vi "PCO_SetRecordingStruct.vi"(8 "error in (no error)":errorcluster {"code" format="%x"}, 10 "strRecording":T1, 11 "ph":u64) -> (0 "error out":errorcluster {"code" format="%x"}, 2 "ErrorMessage":i32 format="%x", 3 "ph out":u64)   [LabVIEW 2019, in "SDK.lvlib" / "RecordingControl.lvlib"]
doc: "<b>Description:</b>\nThis function does set the complete set of recording settings at once. For the sake of clarity it is better to use the functions which change distinct parameter despite changing all settings at once.\nAn invalid value for one of the parameter will result in a failure response message.\nThe command will be rejected, if Recording State is [run], see PCO_GetRecordingState.\n\n<b>Supported camera type:</b>\nAll cameras\n\n<b>Descriptor dependency:</b>\nNone"
uses:
  RecordingControl.lvlib
  Structures/Structures.lvlib
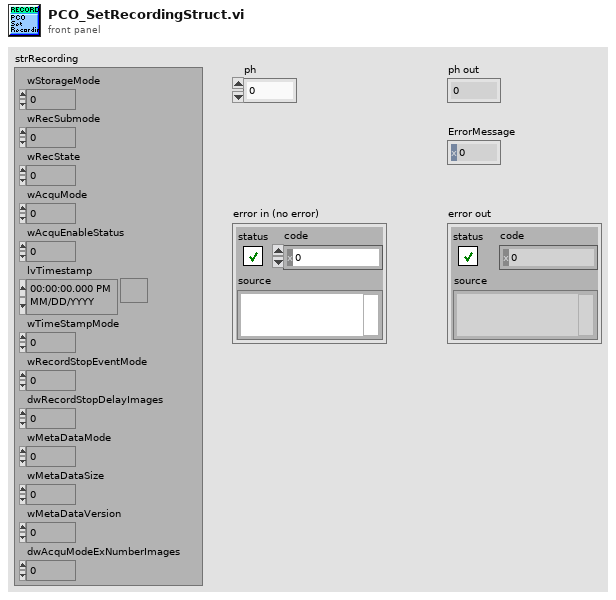
[diagram p1: front panel]
types:
  T1 = cluster{"wStorageMode":u16, "wRecSubmode":u16, "wRecState":u16, "wAcquMode":u16, "wAcquEnableStatus":u16, "lvTimestamp":timestamp, "wTimeStampMode":u16, "wRecordStopEventMode":u16, "dwRecordStopDelayImages":u32, "wMetaDataMode":u16, "wMetaDataSize":u16, "wMetaDataVersion":u16, "dwAcquModeExNumberImages":u32}
  T2 = typedef "LVDateTimeRec.ctl" = cluster{"fractional second":dbl, "second":i32, "minute":i32, "hour":i32, "day of month":i32, "month":i32, "year":i32, "day of week":i32, "day of year":i32, "DST":i32}
  T3 = cluster{"wSize":u16, "wStorageMode":u16, "wRecSubmode":u16, "wRecState":u16, "wAcquMode":u16, "wAcquEnableStatus":u16, "ucDay":u8, "ucMonth":u8, "wYear":u16, "wHour":u16, "ucMin":u8, "ucSec":u8, "wTimeStampMode":u16, "wRecordStopEventMode":u16, "dwRecordStopDelayImages":u32, "wMetaDataMode":u16, "wMetaDataSize":u16, "wMetaDataVersion":u16, "ZZwDummy1":u16, "dwAcquModeExNumberImages":u32, "dwAcquModeExReserved":cluster{u32, u32, u32, u32}, "ZZwDummy":cluster{u16, u16, u16, u16, u16, u16, u16, u16, u16, u16, u16, u16, u16, u16, u16, u16, u16, u16, u16, u16, u16, u16}}
  T4 = cluster{u16, u16, u16, u16, u16, u16, u16, u16, u16, u16, u16, u16, u16, u16, u16, u16, u16, u16, u16, u16, u16, u16}
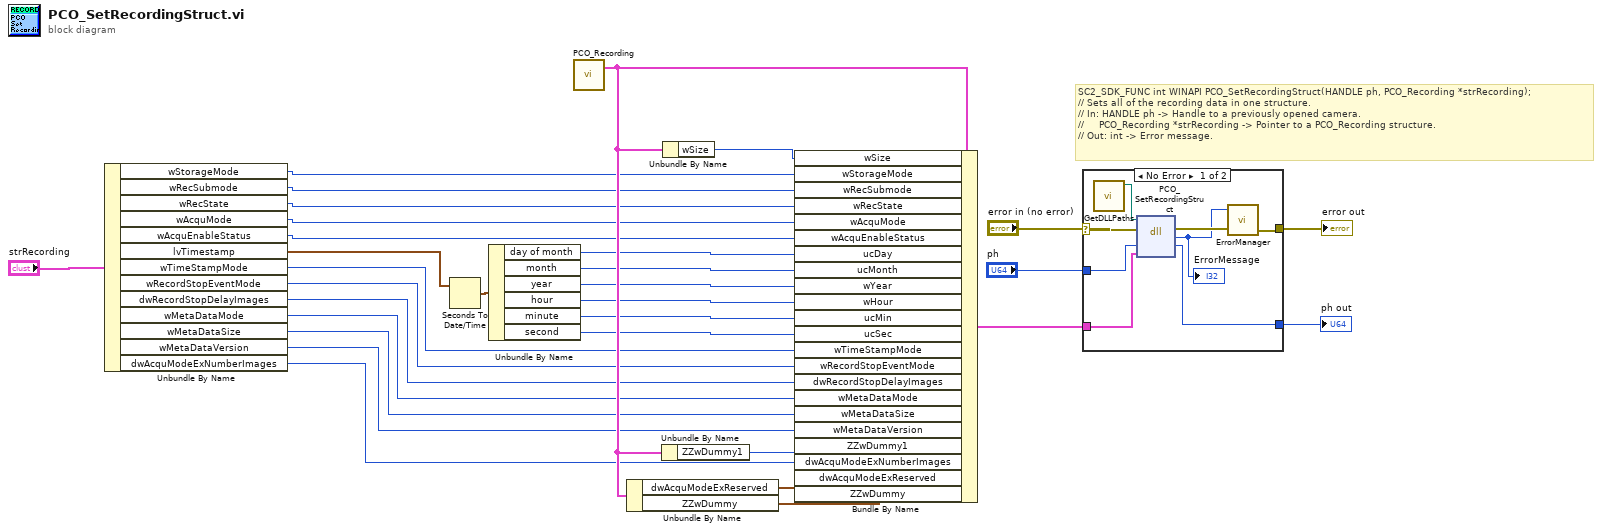
[diagram p0: block diagram]
diagram:
  # "SC2_SDK_FUNC int WINAPI PCO_SetRecordingStruct(HANDLE ph, PCO_Recording *strRecording);\n// Sets all of the recording data in one structure.\n// In: HANDLE ph -> Handle to a previously opened camera.\n//     PCO_Recording *strRecording -> Pointer to a PCO_Recording structure.\n// Out: int -> Error message."
  n1 = Unbundle By Name("strRecording") -> ("wStorageMode"=w18:u16, "wRecSubmode"=w17:u16, "wRecState"=w16:u16, "wAcquMode"=w15:u16, "wAcquEnableStatus"=w14:u16, "lvTimestamp"=w20:timestamp, "wTimeStampMode"=w7:u16, "wRecordStopEventMode"=w6:u16, "dwRecordStopDelayImages"=w5:u32, "wMetaDataMode"=w4:u16, "wMetaDataSize"=w3:u16, "wMetaDataVersion"=w2:u16, "dwAcquModeExNumberImages"=w1:u32)
  n2 = Seconds To Date/Time(time stamp (now)=w20) -> (date time rec=w19:T2)  [unwired: 1 in]
  n3 = Unbundle By Name(w19) -> ("day of month"=w13:i32, "month"=w12:i32, "year"=w11:i32, "hour"=w10:i32, "minute"=w9:i32, "second"=w8:i32)
  n4 = call "PCO_Recording.vi"() -> ("PCO_Recording_Raw"=w25:T3)  [unwired: 4 in, 3 out]
  n5 = Unbundle By Name(w25) -> ("dwAcquModeExReserved"=w24:cluster{u32, u32, u32, u32}, "ZZwDummy"=w23:T4)
  n6 = Unbundle By Name(w25) -> ("ZZwDummy1"=w26:u16)
  n7 = Unbundle By Name(w25) -> ("wSize"=w27:u16)
  n8 = Bundle By Name(cluster=w25, "wSize"=w27, "wStorageMode"=w18, "wRecSubmode"=w17, "wRecState"=w16, "wAcquMode"=w15, "wAcquEnableStatus"=w14, "ucDay"=w13, "ucMonth"=w12, "wYear"=w11, "wHour"=w10, "ucMin"=w9, "ucSec"=w8, "wTimeStampMode"=w7, "wRecordStopEventMode"=w6, "dwRecordStopDelayImages"=w5, "wMetaDataMode"=w4, "wMetaDataSize"=w3, "wMetaDataVersion"=w2, "ZZwDummy1"=w26, "dwAcquModeExNumberImages"=w1, "dwAcquModeExReserved"=w24, "ZZwDummy"=w23) -> (w22:T3)
  n9 = case shown="No Error" "error in (no error)" {
    selector: "error in (no error)" -> [w36 w41]
    tunnel: "ph" -> [w39 w40]
    tunnel: [w38 w40] -> w30
    tunnel: w22 -> [w37 _]
    tunnel: [w34 w41] -> w29
    frame No Error {
      n10 = call "GetDLLPaths.vi"() -> ("SC2_Cam_Path"=w32:path)  [unwired: 8 in, 3 out]
      n11 = dll-call lib="?" fn="PCO_SetRecordingStruct"(path in=w32, error in=w36, "ph"=w39, "strRecording"=w37) -> (error out=w35:errorcluster, "return type"=w33:i32, "ph"=w38:u64)  [unwired: 2 in, 1 out]
      "ErrorMessage" <- w33
      n12 = call "ErrorManager.vi"("error in (no error)"=w35, "error code"=w33) -> ("error out"=w34:errorcluster)  [unwired: 2 in, 1 out]
    }
    frame Error {
    }
  }
  "ph out" <- w30
  "error out" <- w29
